vi "AppleScript Dashboard Setup.vi"(8 "Auto code File path":path, 11 "Automode":i32) -> (1 "Error log":string)   [LabVIEW 2017]
uses:
  <vilib>/Rock Robotics/Network Tables/NT Read String.vi
  <vilib>/Rock Robotics/Network Tables/NT Write String.vi
  <vilib>/Rock Robotics/Network Tables/NT Write Numeric Array.vi
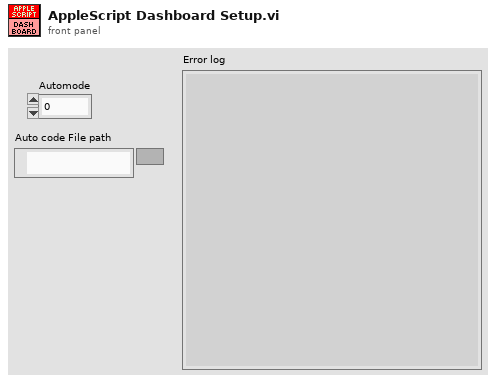
[diagram p1: front panel]
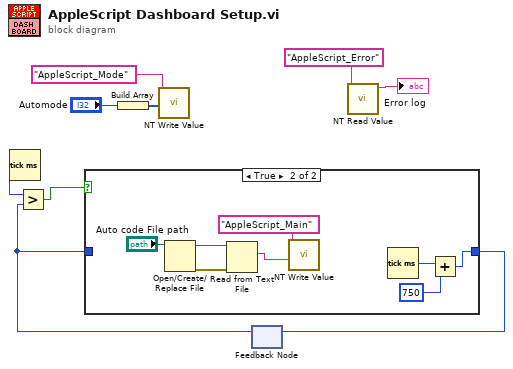
[diagram p0: block diagram]
diagram:
  n1 = Tick Count (ms)() -> (millisecond timer value=w4:u32)
  n2 = Build Array("Automode") -> (w5:i32[])
  n3 = call-poly <vilib>:"NT Write Value.vi"("Numeric Array"=w5, "Name"="AppleScript_Mode") -> ()  [unwired: 9 in, 1 out]
  n4 = feedback #1() -> (w1:u32)  [unwired: 1 in]
  n5 = Greater?(x=w4, y=w1) -> (0:w2:bool)
  n6 = case shown="True" w2 {
    tunnel: [w10 w11] -> w3
    tunnel: w1 -> [w10 _]
    frame False {
    }
    frame True {
      n7 = Open/Create/Replace File(file path (use dialog)="Auto code File path") -> (refnum out=w16:refnum<file>, error out=w17:errorcluster)  [unwired: 5 in, 1 out]
      n8 = Read from Text File(file (use dialog)=w16, error in=w17) -> (text=w15:string)  [unwired: 2 in, 3 out]
      n9 = call-poly <vilib>:"NT Write Value.vi"("String"=w15, "Name"="AppleScript_Main") -> ()  [unwired: 9 in, 1 out]
      n10 = Tick Count (ms)() -> (millisecond timer value=w13:u32)
      n11 = Add(x=w13, y=750) -> (x+y=w11:u32)
    }
  }
  n12 = feedback-in #1(w3) -> ()
  n13 = call-poly <vilib>:"NT Read Value.vi"("Name"="AppleScript_Error") -> ("String"=→"Error log":string)  [unwired: 9 in, 1 out]
